vi "error-生成提示消息.vi"(1 "error in (no error)":errorcluster caption="错误输入（无错误）") -> (0 "错误说明":string)   [LabVIEW 2014]
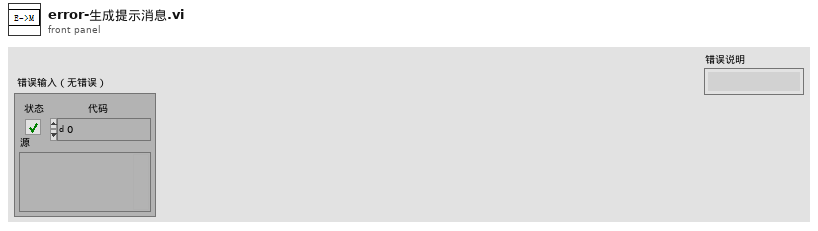
[diagram p1: front panel]
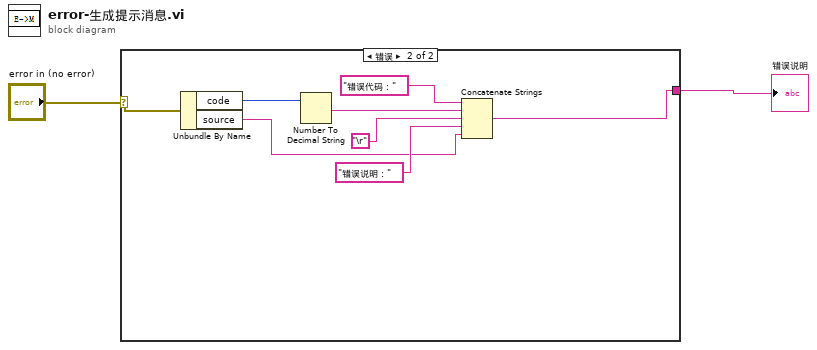
[diagram p0: block diagram]
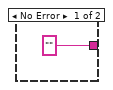
[diagram p2: hidden frame]
diagram:
  n1 = case shown="错误" "error in (no error)" {
    selector: "error in (no error)" -> [_ w11]
    tunnel: ["" w4] -> w1
    frame No Error {
    }
    frame Error {
      n2 = Unbundle By Name(w11) -> ("code"=w10:i32, "source"=w5:string)
      n3 = Number To Decimal String(number=w10) -> (decimal integer string=w9:string)  [unwired: 1 in]
      n4 = Concatenate Strings("错误代码：" ("字符串"), w9, "\r", "错误说明：" ("字符串"), w5) -> (w4:string)
    }
  }
  "错误说明" <- w1
